vi "IMIC_GetZProp.vi"(3 "Enum":T1(ring), 4 "index":i32, 5 "handle":u64) -> (0 "Property":dbl, 1 "handle out":u64, 2 "output param":T2(ring))   [LabVIEW 2011]
uses:
  tillimic32.dll
panel:
  # "never used"
  # "dll not really working here"
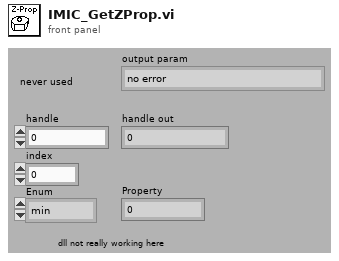
[diagram p1: front panel]
types:
  T1 = enum32{"min", "resolution", "max", "no property"}
  T2 = enum16{"no error", "missing axis", "missing Z axis", "missing Filter", "iMic not initialized", "no property", "wrong handle", "protocol not finished", "user parameter to long (>32 bits)", "no user parameter handle", "failed to open comport", "failed to initialize"}
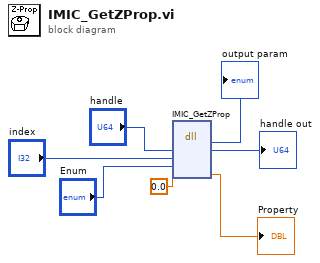
[diagram p0: block diagram]
diagram:
  n1 = dll-call lib="D:/Colibri/Drivers/TILLPhotonics/tillimic*.*" fn="IMIC_GetZProp"("handle"="handle", "index"="index", "propindex"="Enum", "propValue"=0.0) -> ("return type"=→"output param":i32, "handle"=→"handle out":u64, "propValue"=→"Property":dbl)  [unwired: 5 in, 2 out]
